vi "ParseGoalPos.vi"(3 "Old Coords":T1 {"Angle" format="%#_13g"}, 4 "Goal Measurements":dbl[][](array[numeric]), 5 "Camera Angle (Rad)":dbl format="%#_13g") -> (0 "New Coords":T1 {"Angle" format="%#_13g"}, 1 "Target RPM":dbl, 2 "Angle (deg, from vertical)":dbl)   [LabVIEW 2015]
uses:
  <vilib>/Analysis/coordinate.llb/2D Cartesian Coordinate Shift (Scalar).vi
  <vilib>/Analysis/NI_AALPro.lvlib
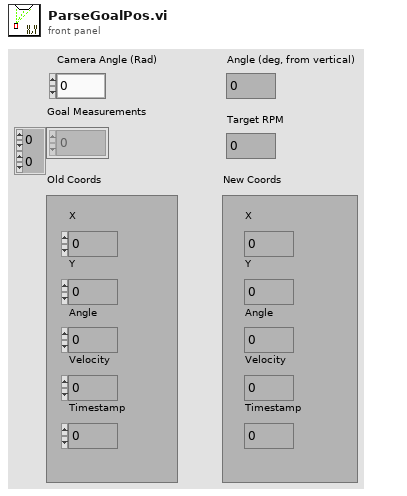
[diagram p1: front panel]
types:
  T1 = cluster{"X":dbl, "Y":dbl, "Angle":dbl, "Velocity":dbl, "Timestamp":u32}
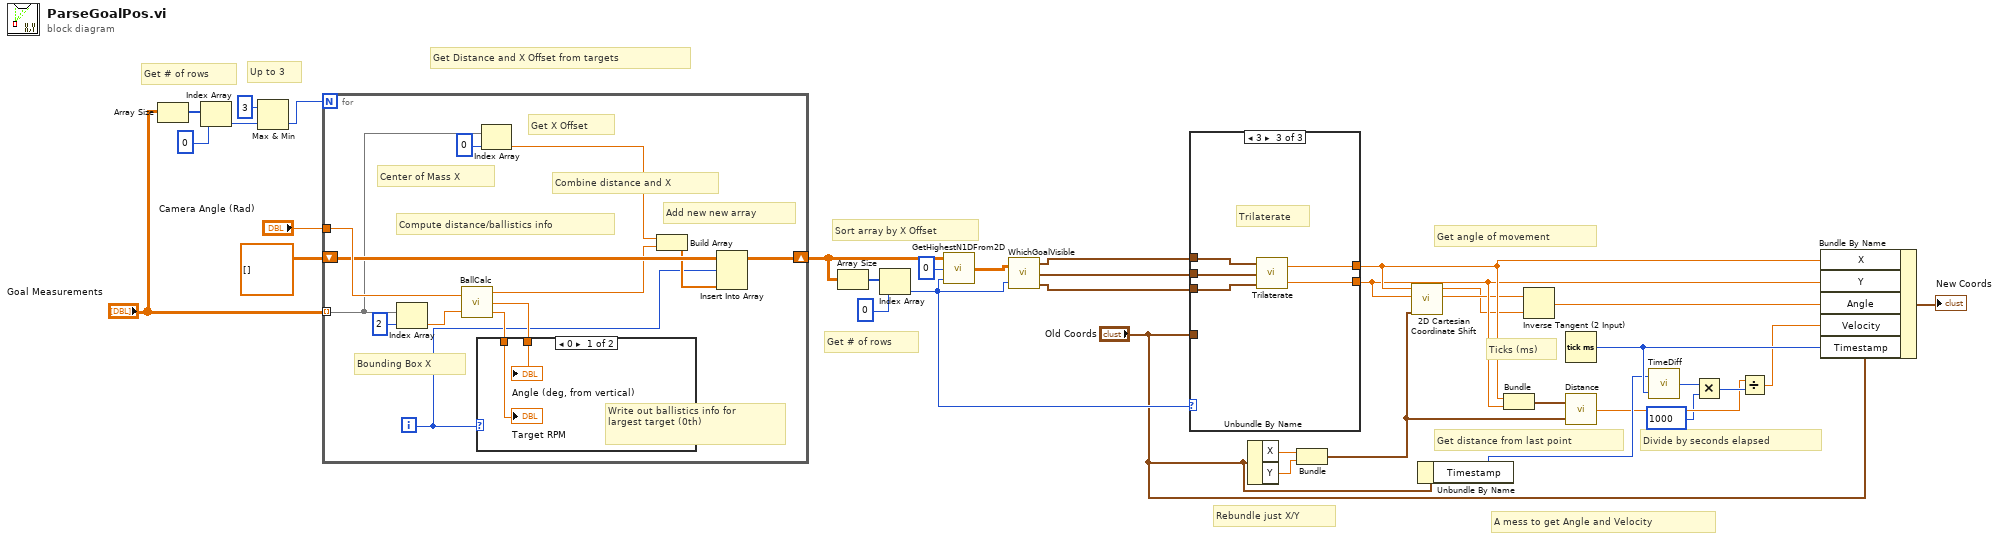
[diagram p0: block diagram]
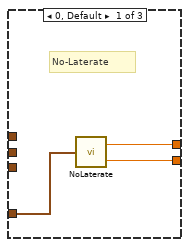
[diagram p2: hidden frame]
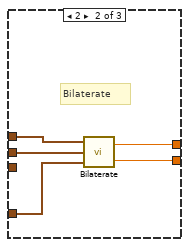
[diagram p3: hidden frame]
diagram:
  # "A mess to get Angle and Velocity"
  # "Get angle of movement"
  # "Ticks (ms)"
  # "Divide by seconds elapsed"
  # "Get distance from last point"
  # "Rebundle just X/Y"
  # "Up to 3"
  # "Get # of rows"
  # "Get # of rows"
  # "Get Distance and X Offset from targets"
  # "Sort array by X Offset"
  n1 = Array Size(array="Goal Measurements") -> (size(s)=w32:i32[])
  n2 = Index Array(array=w32, index=0) -> (element=w25:i32)
  n3 = Max & Min(x=3, y=w25) -> (min(x,y)=w26:i32)  [unwired: 1 out]
  n4 = for {
    N: w26 -> [_]
    tunnel: "Camera Angle (Rad)" -> [w48]
    tunnel: "Goal Measurements" -> [w42] mode=indexing
    shift-right: [w40] -> w27
    shift-left: dbl[][] [] -> [w43]
    i -> [w36]
    # "Add new new array"
    # "Combine distance and X"
    # "Write out ballistics info for\nlargest target (0th)"
    # "Center of Mass X"
    # "Get X Offset"
    # "Compute distance/ballistics info"
    # "Bounding Box X"
    n5 = Index Array(array=w42, index=2) -> (element=w46:dbl)
    n6 = call "BallCalc.vi"("Camera Angle (Rad)"=w48, "Object Viewport Width (px)"=w46) -> ("Target Distance (in)"=w38:dbl, "Angle (deg, from vertical)"=w45:dbl, "Target RPM"=w44:dbl)
    n7 = case shown="0" w36 {
      tunnel: w45 -> [w50 _]
      tunnel: w44 -> [w49 _]
      frame 0 {
        "Angle (deg, from vertical)" <- w50
        "Target RPM" <- w49
      }
      frame 1, Default {
        # "None"
      }
    }
    n8 = Index Array(array=w42, index=0) -> (element=w39:dbl)
    n9 = Build Array(w39, w38) -> (w37:dbl[])
    n10 = Insert Into Array(array=w43, index (row)=w36, new element=w37) -> (w40:dbl[][])  [unwired: 1 in]
  }
  n11 = Array Size(array=w27) -> (size(s)=w29:i32[])
  n12 = Index Array(array=w29, index=0) -> (element=w22:i32)
  n13 = call "GetHighestN1DFrom2D.vi"("# Outputs"=w22, "Sort by Row #"=0, "Array"=w27) -> ("Out"=w23:dbl[][])
  n14 = call "WhichGoalVisible.vi"("Goal Measurements"=w23, "No. of Goals"=w22) -> ("Goal A"=w21:cluster{"X":dbl, "Y":dbl, "Dist":dbl}, "Goal B"=w20:cluster{"X":dbl, "Y":dbl, "Dist":dbl}, "Goal C"=w19:cluster{"X":dbl, "Y":dbl, "Dist":dbl})
  n15 = case shown="3" w22 {
    tunnel: [w53 w58 w60] -> w13
    tunnel: [w52 w57 w59] -> w12
    tunnel: w21 -> [_ w56 w63]
    tunnel: w20 -> [_ w55 w62]
    tunnel: w19 -> [_ _ w61]
    tunnel: "Old Coords" -> [w51 w54 _]
    frame 0, Default {
      # "No-Laterate"
      n16 = call "NoLaterate.vi"("Old Coords"=w51) -> ("x out"=w53:dbl, "y out"=w52:dbl)
    }
    frame 2 {
      # "Bilaterate"
      n17 = call "Bilaterate.vi"("Old"=w54, "B"=w55, "A"=w56) -> ("Y"=w57:dbl, "X"=w58:dbl)
    }
    frame 3 {
      # "Trilaterate"
      n18 = call "Trilaterate.vi"("C"=w61, "B"=w62, "A"=w63) -> ("Y"=w59:dbl, "X"=w60:dbl)
    }
  }
  n19 = Unbundle By Name("Old Coords") -> ("X"=w17:dbl, "Y"=w16:dbl)
  n20 = Bundle("X"=w17, "Y"=w16) -> (w15:cluster{"X":dbl, "Y":dbl})  [unwired: 1 in]
  n21 = call-poly <vilib>:"2D Cartesian Coordinate Shift.vi"("shift"=w15, "y"=w12, "x"=w13) -> ("y out"=w5:dbl, "x out"=w4:dbl)  [unwired: 6 in, 1 out]
  n22 = Unbundle By Name("Old Coords") -> ("Timestamp"=w9:u32)
  n23 = Bundle("X"=w13, "Y"=w12) -> (w14:cluster{"X":dbl, "Y":dbl})  [unwired: 1 in]
  n24 = Inverse Tangent (2 Input)(1:w4, 2:w5) -> (0:w3:dbl)
  n25 = Tick Count (ms)() -> (millisecond timer value=w11:u32)
  n26 = call "Distance.vi"("B"=w15, "A"=w14) -> ("Distance"=w7:dbl)
  n27 = call "TimeDiff.vi"("Time B"=w11, "Time A"=w9) -> ("Time Diff"=w1:u32)
  n28 = Multiply(x=w1, y=u32 1000 ("x")) -> (x*y=w8:u32)
  n29 = Divide(x=w7, y=w8) -> (x/y=w6:dbl)
  n30 = Bundle By Name(cluster="Old Coords", "X"=w13, "Y"=w12, "Angle"=w3, "Velocity"=w6, "Timestamp"=w11) -> (→"New Coords":T1)
